vi "Get Row From Point.vi"(8 "错误输入":errorcluster, 11 "Listbox Ref":refnum<vi>) -> (0 "错误输出":errorcluster, 2 "Point to Row":T1, 3 "Dup Listbox Ref":refnum<vi>)   [LabVIEW 2012, in "Listbox Tool.lvlib"]
uses:
  Listbox Tool.lvlib
  <vilib>/Utility/miscctls.llb/LVPositionTypeDef.ctl
panel:
  in  "Point":T2 caption="点"
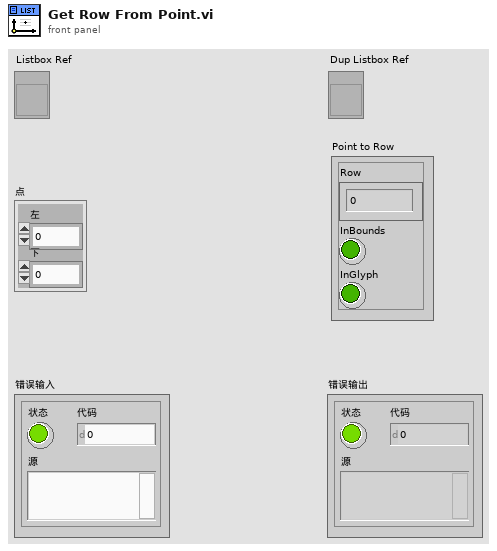
[diagram p1: front panel]
types:
  T1 = cluster{"Row":i32, "InBounds":bool, "InGlyph":bool}
  T2 = typedef "LVPositionTypeDef.ctl" = cluster{"Left":i32, "Top":i32}
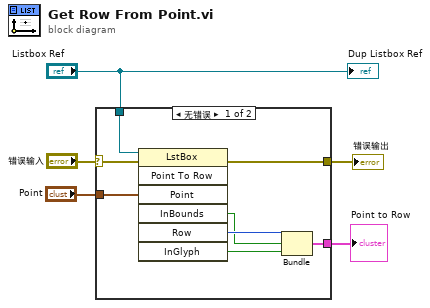
[diagram p0: block diagram]
diagram:
  n1 = case shown="无错误" "错误输入" {
    selector: "错误输入" -> [w10 w14]
    tunnel: "Listbox Ref" -> [w13 _]
    tunnel: [w11 w14] -> w3
    tunnel: "Point" -> [w12 _]
    tunnel: [w6 _] -> w1
    frame No Error {
      n2 = invoke class="LstBox" method="Point To Row"(reference=w13, error in=w10, "Point"=w12) -> (error out=w11:errorcluster, "InBounds"=w8:bool, "Row"=w9:i32, "InGlyph"=w7:bool)  [unwired: 4 in, 3 out]
      n3 = Bundle("Row"=w9, "InBounds"=w8, "InGlyph"=w7) -> (w6:T1)  [unwired: 1 in]
    }
    frame Error {
    }
  }
  "错误输出" <- w3
  "Point to Row" <- w1
  "Dup Listbox Ref" <- "Listbox Ref"
